vi "LLB Pre-Build CHM Build.vi"(6 "Top Level/Always Included VIs":path[](array[path]), 7 "Main Destination Path":path, 9 "Target Name":string, 10 "Build Specification Name":string, 11 "Project Path":path) -> (0 "error out":errorcluster)   [LabVIEW 2017]
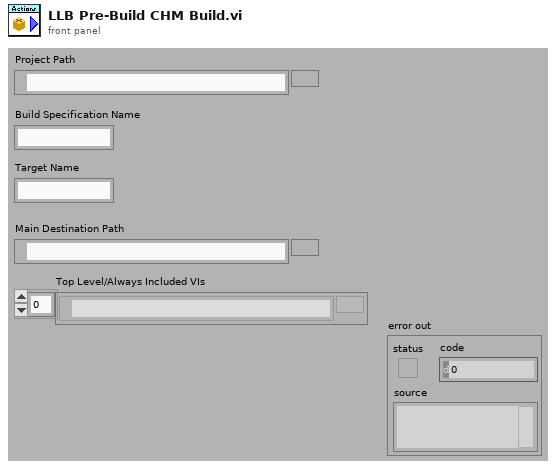
[diagram p1: front panel]
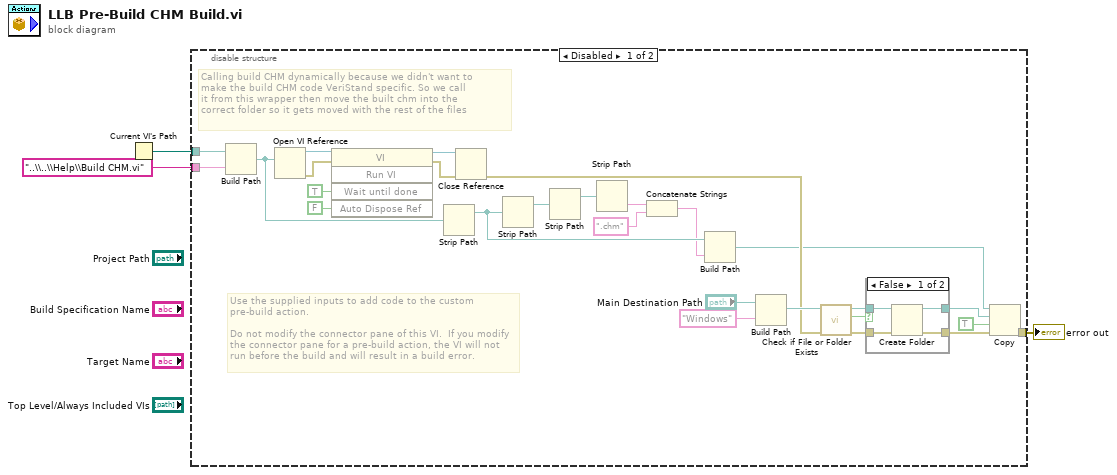
[diagram p0: block diagram]
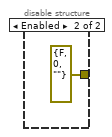
[diagram p3: hidden frame]
diagram:
  n1 = Current VI's Path() -> (path=w3:path)
  n2 = disable-structure shown="Disabled" {
    disable-tunnel: w3 -> [w30 _]
    disable-tunnel: "..\\..\\Help\\Build CHM.vi" ("name or relative path") -> [w29 _]
    disable-tunnel: [w4 errorcluster {"status"=FALSE, "code"=0, "source"=""} ("error out")] -> w1
    frame Disabled {
      # "Calling build CHM dynamically because we didn't want to \nmake the build CHM code VeriStand specific. So we call\nit from this wrapper then move the built chm into the\ncorrect folder so it gets moved with the rest of the files"
      # "Use the supplied inputs to add code to the custom pre-build action.\n\nDo not modify the connector pane of this VI.  If you modify the connector pane for a pre-build action, the VI will not run before the build and will result in a build error."
      n3 = Build Path(base path=w30, name or relative path=w29) -> (appended path=w22:path)
      n4 = Open VI Reference(vi path=w22) -> (vi reference=w28:refnum<vi>, error out=w27:errorcluster)  [unwired: 5 in]
      n5 = invoke class="VI" method="Run VI"(reference=w28, error in=w27, "Wait until done"=TRUE ("Wait Until Done"), "Auto Dispose Ref"=FALSE ("Auto Dispose Reference")) -> (reference out=w24:refnum<vi>, error out=w23:errorcluster)  [unwired: 1 in, 3 out]
      n6 = Strip Path(path=w22) -> (stripped path=w21:path)  [unwired: 1 out]
      n7 = Close Reference(reference=w24, error in (no error)=w23) -> (error out=w12:errorcluster)
      n8 = Strip Path(path=w21) -> (stripped path=w20:path)  [unwired: 1 out]
      n9 = Strip Path(path=w20) -> (stripped path=w19:path)  [unwired: 1 out]
      n10 = Strip Path(path=w19) -> (name=w18:string)  [unwired: 1 out]
      n11 = Concatenate Strings(w18, ".chm" ("string")) -> (w16:string)
      n12 = Build Path(base path=w21, name or relative path=w16) -> (appended path=w5:path)
      n13 = Build Path(base path="Main Destination Path", name or relative path="Windows") -> (appended path=w13:path)
      n14 = call <vilib>:"Check if File or Folder Exists.vi"("error in (no error)"=w12, "path"=w13) -> ("error out"=w9:errorcluster, "file or folder exists?"=w11:bool, "dup path"=w10:path)  [unwired: 7 in]
      n15 = case shown="False" w11 {
        tunnel: w10 -> [w33 w36]
        tunnel: w9 -> [w34 w35]
        tunnel: [w32 w36] -> w7
        tunnel: [w31 w35] -> w8
        frame False {
          n16 = Create Folder(path (use dialog)=w33, error in=w34) -> (created path=w32:path, error out=w31:errorcluster)  [unwired: 1 in, 1 out]
        }
        frame True {
        }
      }
      n17 = Copy(8:w8, 9:TRUE ("overwrite (F)"), 10:w7, 11:w5) -> (0:w4:errorcluster)  [unwired: 1 in, 2 out]
    }
    frame Enabled {
    }
  }
  "error out" <- w1
